vi "Update Linked List Definition.vi"(6 "Unique ID":string, 7 "Parent ID":string, 8 "error in (no error)":errorcluster, 10 "Linked List Definition":refnum<class "Linked List Definition.lvclass">, 11 "Linked List in":refnum<class "Linked List.lvclass">) -> (0 "error out":errorcluster, 3 "Linked List out":refnum<class "Linked List.lvclass">)   [LabVIEW 2020, in "Linked Lists.lvlib" / "Linked List.lvclass"]
uses:
  <vilib>/gpm_packages/@cs/linked-list/Source/Linked List/Linked List/Linked List.lvclass
  <vilib>/gpm_packages/@cs/linked-list/Source/Linked List/Linked List Definition/Linked List Definition.lvclass
  <vilib>/gpm_packages/@cs/linked-list/Source/Linked List/Linked List/Linked List.lvclass/Linked List.ctl
  <vilib>/gpm_packages/@cs/lookup-table/Source/LookupTable/LookupTable.lvclass/LookupTable.ctl
  9da57b77-c7cd-4a51-a2ff-b97e5f401819.vi
  d2a87fe5-5aaf-4518-b2c3-133ef3c660e6.vi
  <vilib>/gpm_packages/@cs/lookup-table/Source/LookupTable/Read Table Reference.vi
  9da57b77-c7cd-4a51-a2ff-b97e5f401819.vi/5a7267ad-595e-4610-9ac2-8bef780848ff.vi
  d2a87fe5-5aaf-4518-b2c3-133ef3c660e6.vi/527409de-c0d9-4f52-b5ac-fa7c64bbfe33.vi
  <vilib>/gpm_packages/@cs/lookup-table/Source/LookupTable/LookupTable.lvclass
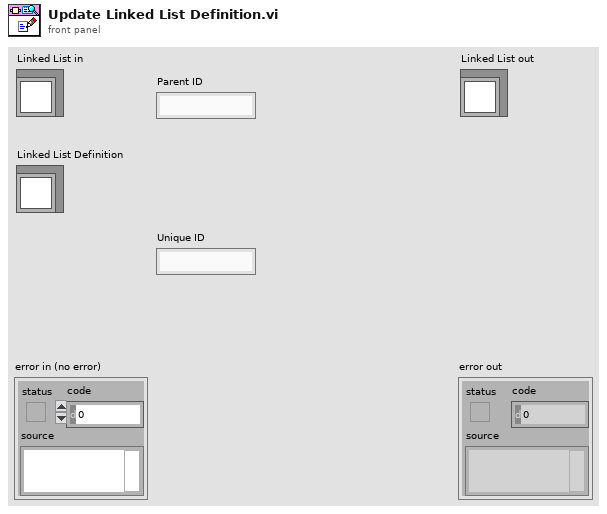
[diagram p1: front panel]
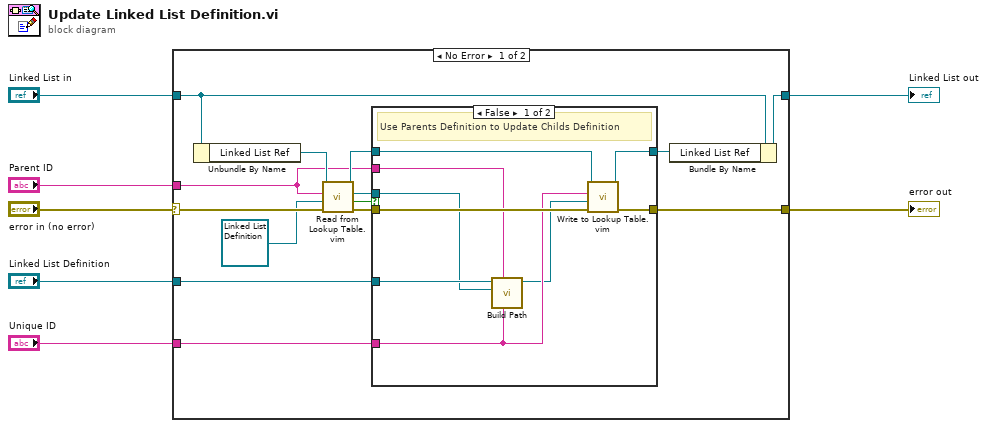
[diagram p0: block diagram]
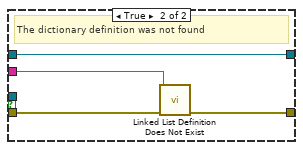
[diagram p2: hidden frame]
diagram:
  n1 = case shown="No Error" "error in (no error)" {
    selector: "error in (no error)" -> [w20 w35]
    tunnel: "Linked List in" -> [w11 w36]
    tunnel: [w14 w35] -> w5
    tunnel: "Parent ID" -> [w13 _]
    tunnel: [w10 w36] -> w6
    tunnel: "Unique ID" -> [w12 _]
    tunnel: "Linked List Definition" -> [w8 _]
    frame No Error {
      n2 = Unbundle By Name(w11) -> ("Linked List Ref"=w21:refnum<data-value>)
      n3 = call "Read from Lookup Table.vim"("error in (no error)"=w20, "Type"=refnum<class "Linked List Definition.lvclass"> refnum ("Linked List.lvlib:Linked List Definition.lvclass"), "Item Name"=w13, "LookupTable Reference"=w21) -> ("error out"=w15:errorcluster, "Not Found?"=w18:bool, "Value"=w16:refnum<class "Linked List Definition.lvclass">, "LookupTable Reference Out"=w17:refnum<data-value>)  [unwired: 4 in]
      n4 = case shown="False" w18 {
        tunnel: w17 -> [w28 w31]
        tunnel: w16 -> [w24 _]
        tunnel: [w29 w33] -> w14
        tunnel: w15 -> [w30 w34]
        tunnel: w13 -> [w25 w32]
        tunnel: w12 -> [w23 _]
        tunnel: [w27 w31] -> w9
        tunnel: w8 -> [w26 _]
        frame False {
          # "Use Parents Definition to Update Childs Definition"
          n5 = call <vilib>:"Build Path.vi"("Unique ID"=w23, "Parent ID"=w25, "Parent Definition"=w24, "Linked List Definition in"=w26) -> ("Linked List Definition out"=w22:refnum<class "Linked List Definition.lvclass">)  [unwired: 6 in, 1 out]
          n6 = call "Write to Lookup Table.vim"("error in (no error)"=w30, "Item"=w22, "Item Name"=w23, "LookupTable Reference"=w28) -> ("error out"=w29:errorcluster, "LookupTable Reference Out"=w27:refnum<data-value>)  [unwired: 5 in, 1 out]
        }
        frame True {
          # "The dictionary definition was not found"
          n7 = call <vilib>:"Linked List Definition Does Not Exist.vi"("Error In"=w34, "Unique ID"=w32) -> ("Error Out"=w33:errorcluster)  [unwired: 9 in]
        }
      }
      n8 = Bundle By Name(cluster=w11, "Linked List Ref"=w9) -> (w10:refnum<class "Linked List.lvclass">)
    }
    frame Error {
    }
  }
  "error out" <- w5
  "Linked List out" <- w6
